vi "CheesyDrive.vi"(6 "Quickturn":bool, 7 "WheelNonLinearity":dbl=0.65, 8 "negInertiaScalar":dbl=1.0, 9 "Sensitivty":dbl=1.0, 10 "Wheel":dbl(slide) scale=-1.0..1.0, 11 "Throttle":dbl(slide)=0.007874015748031496 scale=-1.0..1.0) -> (2 "Right PWM":dbl, 3 "Left PWM":dbl)   [LabVIEW 2017]
doc: "Implements CheesyDrive. CheesyDrive means that the turn joystick controls the radius of turning instead of the rate of turning. Also implements QuickStop and QuickTurn."
panel:
  in  "CarLikeTurning":bool
  in  "QSMult":dbl=0.5
  in  "Max dx/dt":dbl=7.0
  in  "alpha":dbl=0.1
  out "Waveform Chart":dbl(graph)
  # "Enable to enable"
  # "(for quickstop decay)"
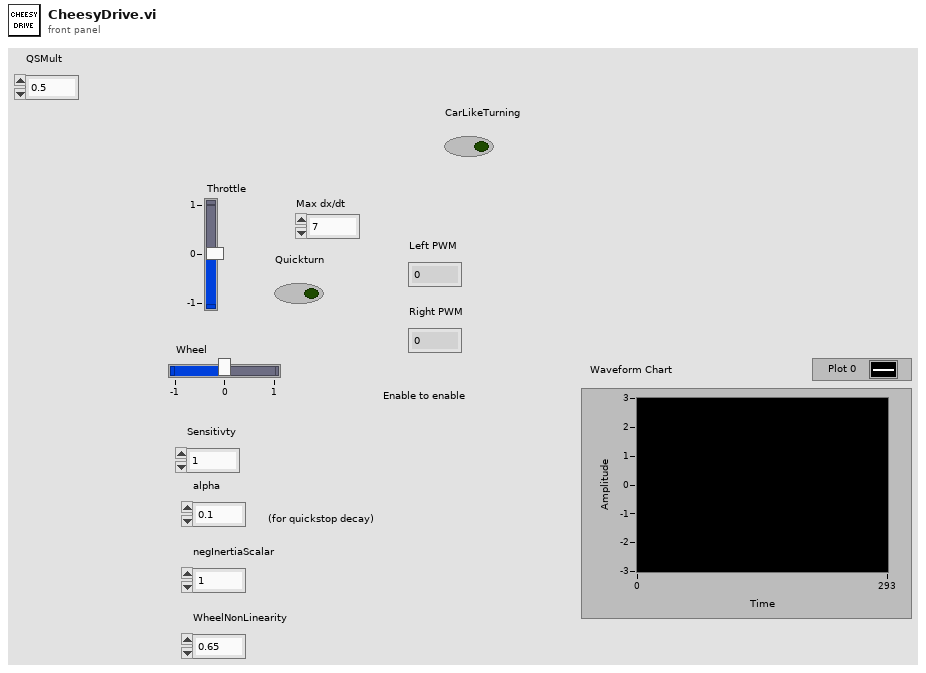
[diagram p1: front panel]
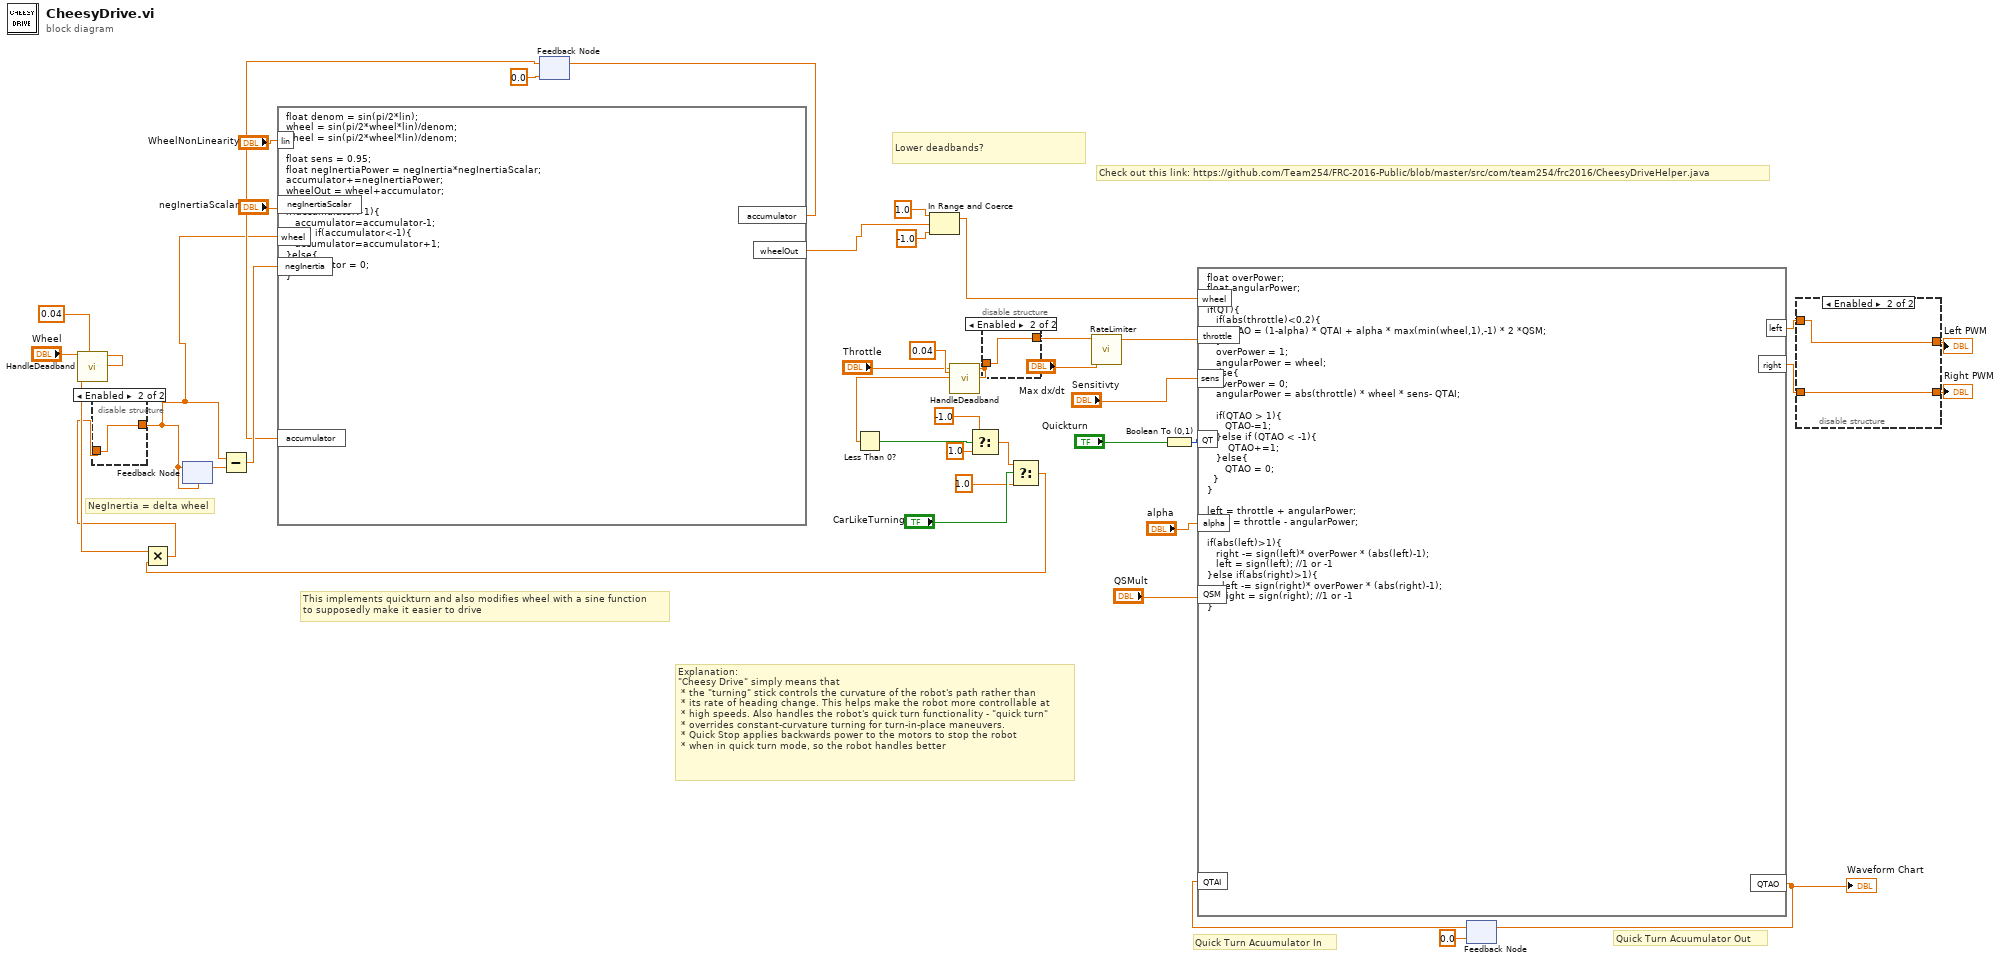
[diagram p0: block diagram]
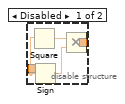
[diagram p2: hidden frame]
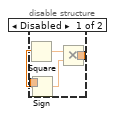
[diagram p3: hidden frame]
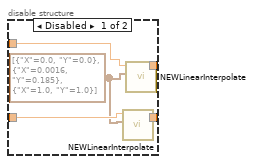
[diagram p4: hidden frame]
diagram:
  # "This implements quickturn and also modifies wheel with a sine function\nto supposedly make it easier to drive"
  # "Lower deadbands?"
  # "NegInertia = delta wheel"
  # "Explanation:\n\"Cheesy Drive\" simply means that\n * the \"turning\" stick controls the curvature of the robot's path rather than\n * its rate of heading change. This helps make the robot more controllable at\n * high speeds. Also handles the robot's quick turn functionality - \"quick turn\"\n * overrides constant-curvature turning for turn-in-place maneuvers.\n * Quick Stop applies backwards power to the motors to stop the robot\n * when in quick turn mode, so the robot handles better"
  # "Quick Turn Acuumulator Out"
  # "Quick Turn Acuumulator In"
  # "Check out this link: https://github.com/Team254/FRC-2016-Public/blob/master/src/com/team254/frc2016/CheesyDriveHelper.java"
  n1 = call "HandleDeadband.vi"("Deadband"=0.04, "Input"="Wheel") -> ("Output"=w7:dbl)  [unwired: 9 in]
  n2 = feedback #1(0.0 ("Wheel")) -> (w23:dbl)
  n3 = call "HandleDeadband.vi"("Deadband"=0.04, "Input"="Throttle") -> ("Output"=w8:dbl)  [unwired: 9 in]
  n4 = Less Than 0?(x=w8) -> (x < 0?=w11:bool)
  n5 = Select(t=-1.0, s=w11, f=1.0) -> (s? t:f=w3:dbl)
  n6 = disable-structure shown="Enabled" {
    disable-tunnel: [w43 w46] -> w32
    disable-tunnel: w8 -> [w42 w46]
    frame Disabled {
      n7 = Square(x=w42) -> (x^2=w45:dbl)
      n8 = Sign(1:w42) -> (0:w44:dbl)
      n9 = Multiply(x=w45, y=w44) -> (x*y=w43:dbl)
    }
    frame Enabled {
    }
  }
  n10 = Select(t=w3, s="CarLikeTurning", f=1.0) -> (s? t:f=w1:dbl)
  n11 = Multiply(x=w7, y=w1) -> (x*y=w6:dbl)
  n12 = disable-structure shown="Enabled" {
    disable-tunnel: w6 -> [w48 w51]
    disable-tunnel: [w47 w51] -> w5
    frame Disabled {
      n13 = Square(x=w48) -> (x^2=w50:dbl)
      n14 = Sign(1:w48) -> (0:w49:dbl)
      n15 = Multiply(x=w50, y=w49) -> (x*y=w47:dbl)
    }
    frame Enabled {
    }
  }
  n16 = feedback #2(w5) -> (w25:dbl)
  n17 = feedback-in #2(w5) -> ()
  n18 = Subtract(x=w5, y=w25) -> (x-y=w24:dbl)
  n19 = formula code="float denom = sin(pi/2*lin);\nwheel = sin(pi/2*wheel*lin)/denom;\nwheel = sin(pi/2*wheel*lin)/denom;\n\nfloat sens = 0.95;\nfloat negInertiaPower = negInertia*negInertiaScalar;\naccumulator+=negInertiaPower;\nwheelOut = wheel+accumulator;\n\nif(accumulator>1){\n   accumulator=accumulator-1;\n}else if(accumulator<-1){\n   accumulator=accumulator+1;\n}else{\naccumulator = 0;\n}"("wheel"=w5, "negInertia"=w24, "accumulator"=w23, "negInertiaScalar"="negInertiaScalar", "lin"="WheelNonLinearity") -> ("accumulator"=w21:dbl, "wheelOut"=w15:dbl)
  n20 = feedback-in #1(w21) -> ()
  n21 = In Range and Coerce(upper limit=1.0, x=w15, lower limit=-1.0) -> (coerced(x)=w16:dbl)  [unwired: 1 out]
  n22 = call "RateLimiter.vi"("Max dx/dt"="Max dx/dt", "Input"=w32) -> ("Output"=w31:dbl)  [unwired: 9 in]
  n23 = Boolean To (0,1)(Boolean="Quickturn") -> (0, 1=w36:i16)
  n24 = feedback #3(0.0 ("QTAccumulatorO")) -> (w34:dbl)
  n25 = formula code="float overPower;\nfloat angularPower;\n\nif(QT){\n   if(abs(throttle)<0.2){\n      QTAO = (1-alpha) * QTAI + alpha * max(min(wheel,1),-1) * 2 *QSM;\n   }\n   overPower = 1;\n   angularPower = wheel;\n}else{\n   overPower = 0;\n   angularPower = abs(throttle) * wheel * sens- QTAI;\n\n   if(QTAO > 1){\n      QTAO-=1;\n   }else if (QTAO < -1){\n       QTAO+=1;\n   }else{\n      QTAO = 0;\n  }\n}\n\nleft = throttle + angularPower;\nright = throttle - angularPower;\n\nif(abs(left)>1){\n   right -= sign(left)* overPower * (abs(left)-1);\n   left = sign(left); //1 or -1\n}else if(abs(right)>1){\n     left -= sign(right)* overPower * (abs(right)-1);\n     right = sign(right); //1 or -1 \n}"("wheel"=w16, "throttle"=w31, "sens"="Sensitivty", "QT"=w36, "alpha"="alpha", "QTAI"=w34, "QSM"="QSMult") -> ("left"=w29:dbl, "right"=w26:dbl, "QTAO"=w37:dbl)
  "Waveform Chart" <- w37
  n26 = feedback-in #3(w37) -> ()
  n27 = disable-structure shown="Enabled" {
    disable-tunnel: w29 -> [w56 w58]
    disable-tunnel: [w55 w58] -> w28
    disable-tunnel: [w54 w57] -> w27
    disable-tunnel: w26 -> [w53 w57]
    frame Disabled {
      w52 = cluster{"X":dbl, "Y":dbl}[] [{"X"=0.0, "Y"=0.0}, {"X"=0.0016, "Y"=0.185}, {"X"=1.0, "Y"=1.0}] ("Points")
      n28 = call "NEWLinearInterpolate.vi"("Points"=w52, "Value"=w53) -> ("Output"=w54:dbl)  [unwired: 9 in]
      n29 = call "NEWLinearInterpolate.vi"("Points"=w52, "Value"=w56) -> ("Output"=w55:dbl)  [unwired: 9 in]
    }
    frame Enabled {
    }
  }
  "Left PWM" <- w28
  "Right PWM" <- w27
